vi "top vi.vi"() -> ()   [LabVIEW 2014]
panel:
  in  "開始":bool
  in  "得分":dbl
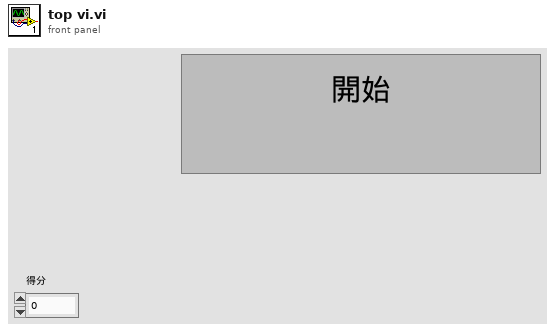
[diagram p1: front panel]
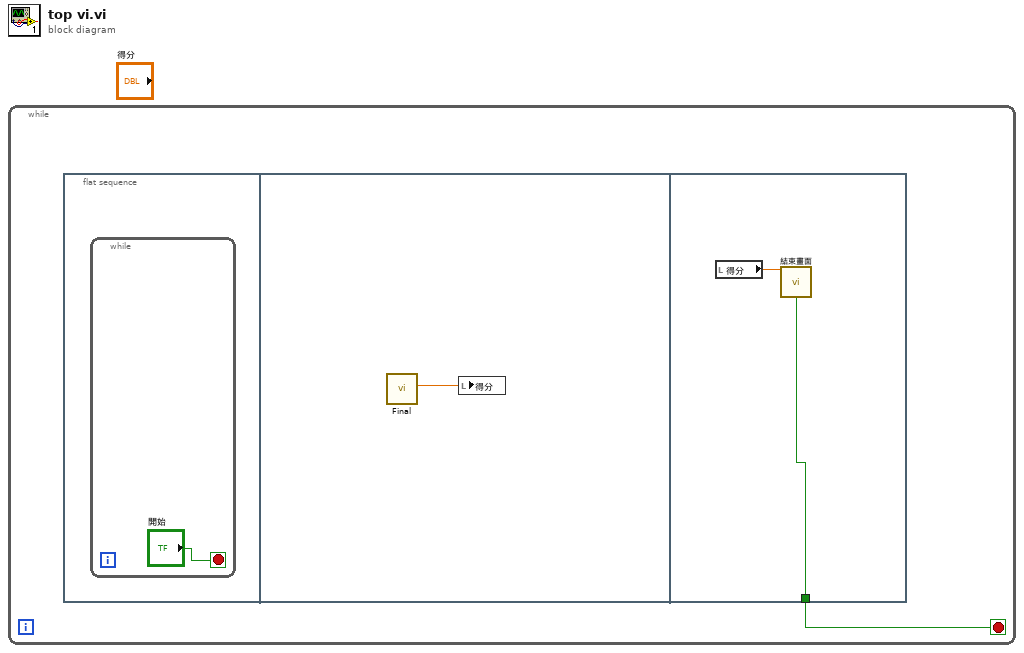
[diagram p0: block diagram]
diagram:
  n1 = while {
    stop <- w1 stop-if-true
    n2 = flat-sequence {
      tunnel: [w5] -> w1
      frame #0 {
        n3 = while {
          stop <- "開始" stop-if-true
        }
      }
      frame #1 {
        n4 = call "Final.vi"() -> ("輸出分數"=w3:dbl)  [unwired: 3 in]
        n5 = local write "得分"(w3) -> ()
      }
      frame #2 {
        n6 = local read "得分"() -> (w4:dbl)
        n7 = call "結束畫面.vi"("Numeric"=w4) -> ("結束遊戲 2"=w5:bool)  [unwired: 1 out]
      }
    }
  }
